vi "test_Basic Host Api.vi"(8 "error in (no error)":errorcluster, 11 "TestCase in":refnum<class "Instrument Addon Host API Tests.lvclass">) -> (0 "error out":errorcluster, 3 "TestCase out":refnum<class "Instrument Addon Host API Tests.lvclass">)   [LabVIEW 2019, in "Instrument Addon Host API Tests.lvclass"]
uses:
  Instrument Addon Host API Tests.lvclass
  Addon/Addon Shared/Types/Buffered RT Instrument Command.ctl
  Addon/Addon Shared/Types/Response Wait Type.ctl
  <vilib>/addons/_JKI Toolkits/VI Tester/TestCase.llb/TestCase.lvclass
  APIs/Host Automation API/Instrument Host Automation API.lvlib
  Addon/Addon Shared/Instrument Addon Shared.lvlib
  C:/Program Files (x86)/National Instruments/LabVIEW 2019/vi.lib/NI/VeriStand Custom Device Testing Tools/VeriStandTestCase/VeriStandTestCase.lvclass
  C:/Program Files (x86)/National Instruments/LabVIEW 2019/vi.lib/addons/_JKI Toolkits/VI Tester/TestCase.llb/TestCase.lvclass
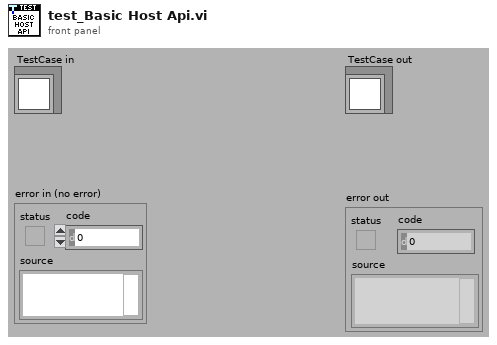
[diagram p1: front panel]
types:
  T1 = typedef "Instrument Addon Shared.lvlib/Buffered RT Instrument Command.ctl" = cluster{"Command":string, "Response Expected?":bool, "Wait Type":T2, "Wait Value":dbl}
  T2 = typedef "Instrument Addon Shared.lvlib/Response Wait Type.ctl" = enum16{"Byte Count", "Wait sec"}
  T3 = typedef "NI STM.lvlib/TCP Connection Info.ctl" = cluster{"connection ID":refnum<k5>, "meta data":T4[]}
  T4 = typedef "NI STM.lvlib/MetaDataElement.ctl" = string
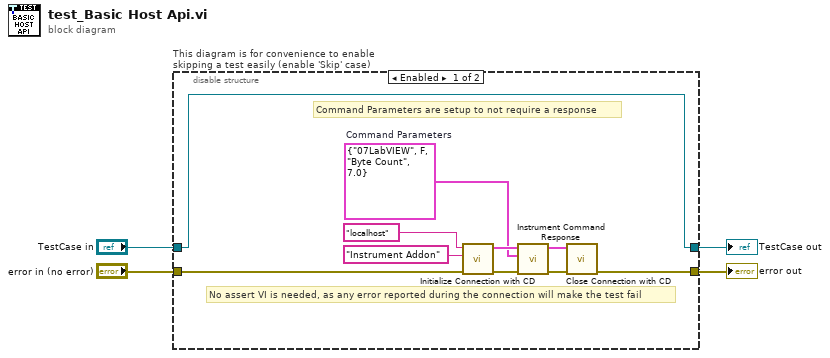
[diagram p0: block diagram]
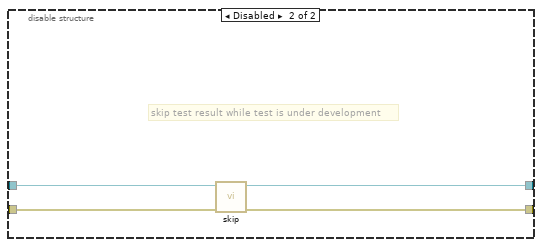
[diagram p2: hidden frame]
diagram:
  n1 = disable-structure "This diagram is for convenience to enable skipping a test easily (enable 'Skip' case)" shown="Enabled" {
    disable-tunnel: "TestCase in" -> [w6 w18]
    disable-tunnel: [w6 w16] -> w1
    disable-tunnel: [w5 w17] -> w3
    disable-tunnel: "error in (no error)" -> [w7 w15]
    frame Enabled {
      w10 = T1 {"Command"="07LabVIEW", "Response Expected?"=FALSE, "Wait Type"=enum."Byte Count", "Wait Value"=7.0}  # Command Parameters
      # "Command Parameters are setup to not require a response"
      # "No assert VI is needed, as any error reported during the connection will make the test fail"
      n2 = call "Initialize Connection with CD.vi"("error in (no error)"=w7, "TCP Service"="Instrument Addon", "IP Address"="localhost") -> ("error out"=w12:errorcluster, "connection info out"=w11:T3)  [unwired: 7 in]
      n3 = call "Instrument Command Response.vi"("error in (no error)"=w12, "Command Parameters"=w10, "Comm.Info"=w11) -> ("error out"=w8:errorcluster, "Comm.Info"=w9:T3)  [unwired: 5 in, 2 out]
      n4 = call "Close Connection with CD.vi"("error in"=w8, "Comm.Info"=w9) -> ("error out"=w5:errorcluster)  [unwired: 9 in]
    }
    frame Disabled {
      # "skip test result while test is under development"
      n5 = call <vilib>:"skip.vi"("error in (no error)"=w15, "TestCase in"=w18) -> ("error out"=w17:errorcluster, "TestCase out"=w16:refnum<class "Instrument Addon Host API Tests.lvclass">)  [unwired: 8 in]
    }
  }
  "error out" <- w3
  "TestCase out" <- w1
